vi "append_temp_probe.vi"(8 "error in (no error)":errorcluster, 10 "TempProbe in":refnum<class "TempProbe.lvclass">, 11 "TempProbeSet in":refnum<class "TempProbeSet.lvclass">) -> (0 "error out":errorcluster, 3 "TempProbeSet out":refnum<class "TempProbeSet.lvclass">)   [LabVIEW 2010, in "TempProbeSet.lvclass"]
uses:
  TempProbeSet.lvclass
  TempProbe.lvclass
  TempProbeSet.lvclass/TempProbeSet.ctl
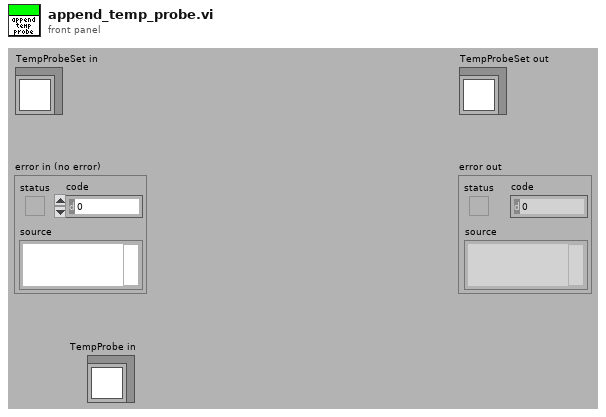
[diagram p1: front panel]
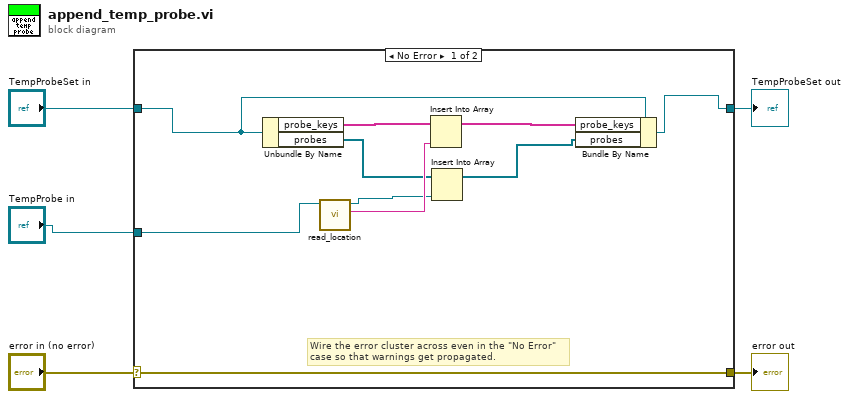
[diagram p0: block diagram]
diagram:
  n1 = case shown="No Error" "error in (no error)" {
    selector: "error in (no error)" -> [w15 w17]
    tunnel: [w15 w17] -> w4
    tunnel: [w14 w16] -> w2
    tunnel: "TempProbeSet in" -> [w12 w16]
    tunnel: "TempProbe in" -> [w13 _]
    frame No Error {
      # "Wire the error cluster across even in the \"No Error\"\ncase so that warnings get propagated."
      n2 = Unbundle By Name(w12) -> ("probe_keys"=w11:string[], "probes"=w8:refnum<class "TempProbe.lvclass">[])
      n3 = call-dynamic "read_location.vi"("TempProbe in"=w13) -> ("Location"=w9:string, "TempProbe out"=w6:refnum<class "TempProbe.lvclass">)  [unwired: 8 in, 1 out]
      n4 = Insert Into Array(array=w11, new element=w9) -> (w10:string[])  [unwired: 1 in]
      n5 = Insert Into Array(array=w8, new element=w6) -> (w7:refnum<class "TempProbe.lvclass">[])  [unwired: 1 in]
      n6 = Bundle By Name(cluster=w12, "probe_keys"=w10, "probes"=w7) -> (w14:refnum<class "TempProbeSet.lvclass">)
    }
    frame Error {
    }
  }
  "error out" <- w4
  "TempProbeSet out" <- w2
